vi "AlliGator Get Phasor Ratio Map Color v3.vi"(7 "Color Fading?":bool, 8 "Error In":errorcluster, 9 "Pixel Color":T1, 10 "-d_0":sgl, 11 "Phasor Ratio Data":T2) -> (0 "Error Out":errorcluster, 1 "Transparent?":bool, 3 "Overlay Color":T1)   [LabVIEW 2021, in "AlliGator Phasor Ratio.lvlib"]
doc: "Computes phasor ratio equivalent color using the provided color scale."
uses:
  AlliGator Phasor Ratio.lvlib
  AlliGator Phasor Ratio Data.ctl
panel:
  # "see the AlliGator License on the block diagram (Ctrl+E or Window:Show Block Diagram)"
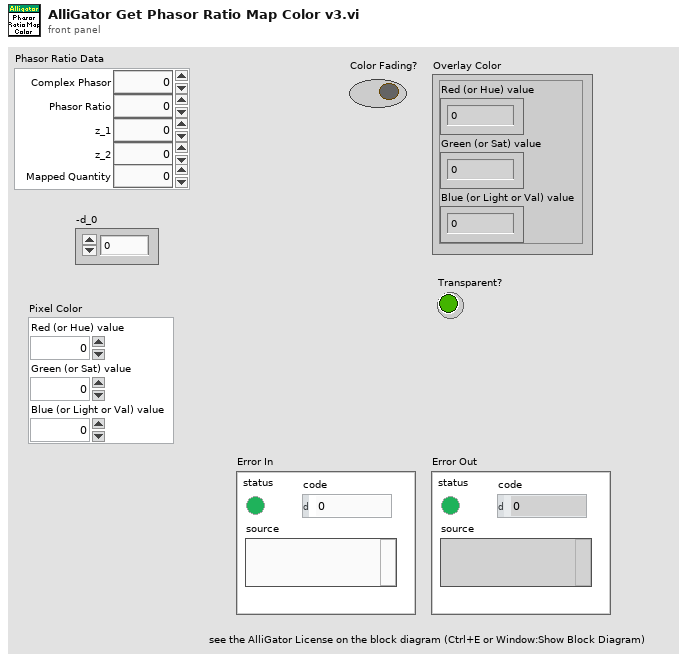
[diagram p1: front panel]
types:
  T1 = cluster{"Red (or Hue) value":u8, "Green (or Sat) value":u8, "Blue (or Light or Val) value":u8}
  T2 = typedef "AlliGator Phasor Ratio.lvlib/AlliGator Phasor Ratio Data.ctl" = cluster{"Complex Phasor":csg, "Phasor Ratio":sgl, "z_1":csg, "z_2":csg, "Mapped Quantity":sgl}
  T3 = cluster{"Red (or Hue) value":sgl, "Green (or Sat) value":sgl, "Blue (or Light or Val) value":sgl}
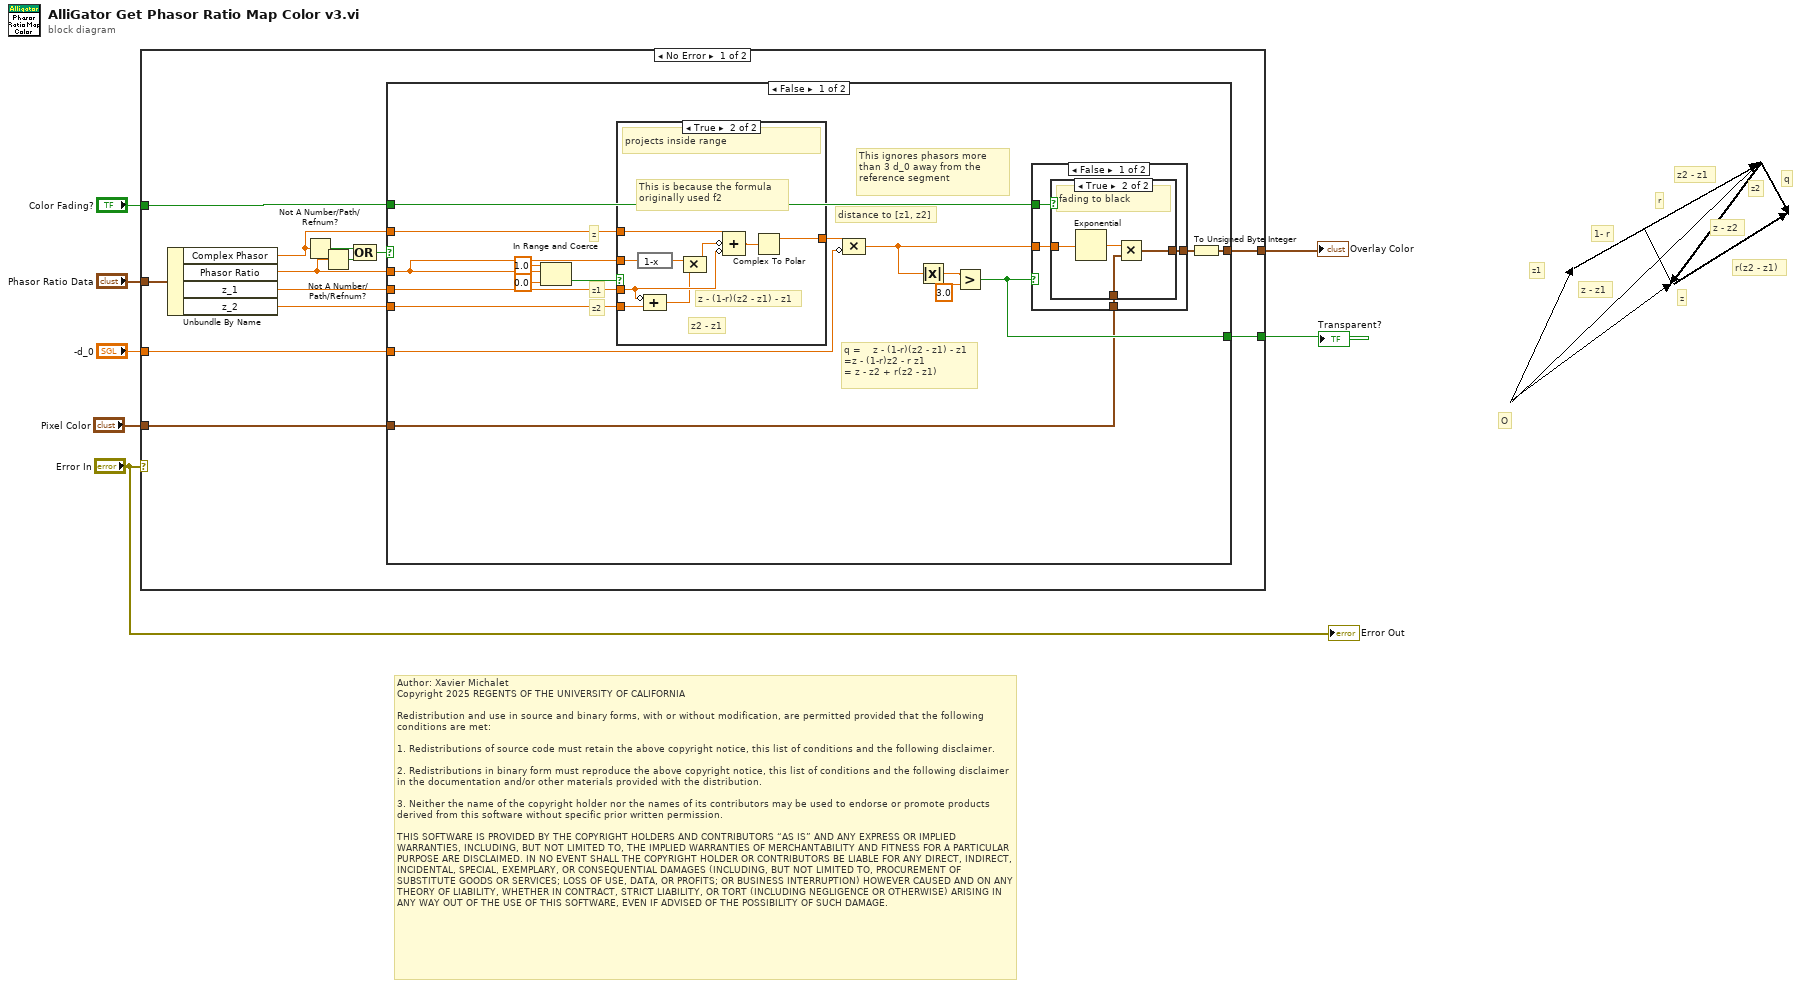
[diagram p0: block diagram]
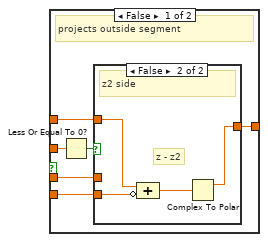
[diagram p4: hidden frame]
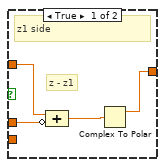
[diagram p5: hidden frame]
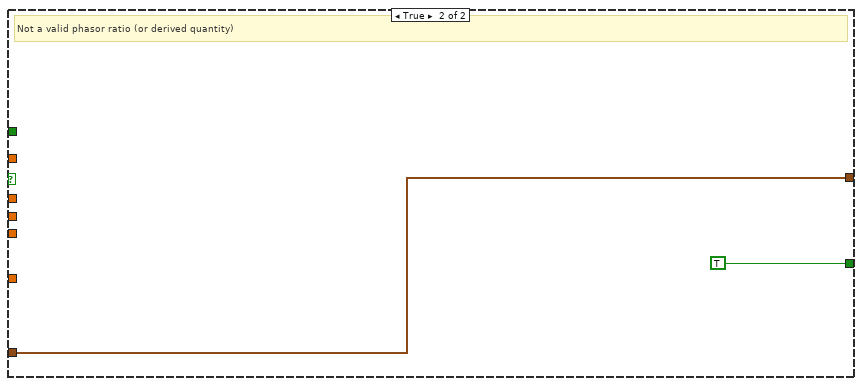
[diagram p6: hidden frame]
diagram:
  # "Author: Xavier Michalet\nCopyright 2025 REGENTS OF THE UNIVERSITY OF CALIFORNIA\n\nRedistribution and use in source and binary forms, with or without modification, are permitted provided that the following conditions are met:\n\n1. Redistributions of source code must retain the above copyright notice, this list of conditions and the following disclaimer.\n\n2. Redistributions in binary form must reproduce the above copyright notice, this list of conditions and the following disclaimer in the documentation and/or other materials provided with the distribution.\n\n3. Neither the name of the copyright holder nor the names of its contributors may be used to endorse or promote products derived from this software without specific prior written permission.\n\nTHIS SOFTWARE IS PROVIDED BY THE COPYRIGHT HOLDERS AND CONTRIBUTORS “AS IS” AND ANY EXPRESS OR IMPLIED WARRANTIES, INCLUDING, BUT NOT LIMITED TO, THE IMPLIED WARRANTIES OF MERCHANTABILITY AND FITNESS FOR A PARTICULAR PURPOSE ARE DISCLAIMED. IN NO EVENT SHALL THE COPYRIGHT HOLDER OR CONTRIBUTORS BE LIABLE FOR ANY DIRECT, INDIRECT, INCIDENTAL, SPECIAL, EXEMPLARY, OR CONSEQUENTIAL DAMAGES (INCLUDING, BUT NOT LIMITED TO, PROCUREMENT OF SUBSTITUTE GOODS OR SERVICES; LOSS OF USE, DATA, OR PROFITS; OR BUSINESS INTERRUPTION) HOWEVER CAUSED AND ON ANY THEORY OF LIABILITY, WHETHER IN CONTRACT, STRICT LIABILITY, OR TORT (INCLUDING NEGLIGENCE OR OTHERWISE) ARISING IN ANY WAY OUT OF THE USE OF THIS SOFTWARE, EVEN IF ADVISED OF THE POSSIBILITY OF SUCH DAMAGE."
  # "O"
  # "q"
  # "r(z2 - z1)"
  # "1- r"
  # "r"
  # "z - z2"
  # "z - z1"
  # "z2 - z1"
  # "z"
  # "z2"
  # "z1"
  n1 = case shown="No Error" "Error In" {
    tunnel: "-d_0" -> [w20 _]
    tunnel: [w19 _] -> w6
    tunnel: [w18 _] -> w5
    tunnel: "Color Fading?" -> [w17 _]
    tunnel: "Phasor Ratio Data" -> [w13 _]
    tunnel: "Pixel Color" -> [w8 _]
    frame No Error {
      n2 = Unbundle By Name(w13) -> ("Complex Phasor"=w12:csg, "Phasor Ratio"=w11:sgl, "z_1"=w10:csg, "z_2"=w9:csg)
      n3 = Not A Number/Path/Refnum?(number/path/refnum=w12) -> (NaN/Path/Refnum?=w16:bool)
      n4 = Not A Number/Path/Refnum?(number/path/refnum=w11) -> (NaN/Path/Refnum?=w15:bool)
      n5 = Compound Arithmetic op=OR(w16, w15) -> (w14:bool)
      n6 = case shown="False" w14 {
        tunnel: w10 -> [w37 _]
        tunnel: w9 -> [w36 _]
        tunnel: w20 -> [w34 _]
        tunnel: [w29 w71] -> w19
        tunnel: [w32 TRUE] -> w18
        tunnel: w17 -> [w31 _]
        tunnel: w12 -> [w30 _]
        tunnel: w11 -> [w28 _]
        tunnel: w8 -> [w21 w71]
        frame False {
          # "distance to [z1, z2]"
          # "q =    z - (1-r)(z2 - z1) - z1\n=z - (1-r)z2 - r z1\n= z - z2 + r(z2 - z1)"
          # "z"
          # "z2"
          # "z1"
          # "This ignores phasors more than 3 d_0 away from the reference segment"
          n7 = In Range and Coerce(upper limit=sgl 1.0, x=w28, lower limit=sgl 0.0) -> (In Range?=w27:bool)  [unwired: 1 out]
          n8 = case shown="True" w27 {
            tunnel: w30 -> [w51 w70]
            tunnel: w37 -> [w50 w64]
            tunnel: w28 -> [w53 w69]
            tunnel: [w49 w66] -> w35
            tunnel: w36 -> [w48 w65]
            frame False {
              # "projects outside segment"
              n9 = Less Or Equal To 0?(x=w53) -> (x <= 0?=w52:bool)
              n10 = case shown="False" w52 {
                tunnel: w51 -> [w57 w61]
                tunnel: w50 -> [w56 _]
                tunnel: [w54 w59] -> w49
                tunnel: w48 -> [_ w58]
                frame True {
                  # "z - z1"
                  # "z1 side"
                  n11 = Compound Arithmetic op=ADD(w57, invert w56) -> (w55:csg)
                  n12 = Complex To Polar(r * e^(i*theta)=w55) -> (r=w54:sgl)  [unwired: 1 out]
                }
                frame False {
                  # "z - z2"
                  # "z2 side"
                  n13 = Compound Arithmetic op=ADD(w61, invert w58) -> (w60:csg)
                  n14 = Complex To Polar(r * e^(i*theta)=w60) -> (r=w59:sgl)  [unwired: 1 out]
                }
              }
            }
            frame True {
              # "z - (1-r)(z2 - z1) - z1"
              # "z2 - z1"
              # "This is because the formula originally used f2"
              # "projects inside range"
              n15 = expression code="1-x"(w69) -> (w62:sgl)
              n16 = Compound Arithmetic op=ADD(invert w64, w65) -> (w63:csg)
              n17 = Compound Arithmetic op=MULTIPLY(w62, w63) -> (w68:csg)
              n18 = Compound Arithmetic op=ADD(w70, invert w68, invert w64) -> (w67:csg)
              n19 = Complex To Polar(r * e^(i*theta)=w67) -> (r=w66:sgl)  [unwired: 1 out]
            }
          }
          n20 = Compound Arithmetic op=MULTIPLY(w35, invert w34) -> (w24:sgl)
          n21 = Absolute Value(x=w24) -> (abs(x)=w23:sgl)
          n22 = Greater?(x=w23, y=sgl 3.0) -> (0:w32:bool)
          n23 = case shown="False" w32 {
            tunnel: w21 -> [w41 w47]
            tunnel: w24 -> [w40 _]
            tunnel: [w39 w47] -> w33
            tunnel: w31 -> [w38 _]
            frame False {
              n24 = case shown="True" w38 {
                tunnel: w41 -> [w42 w46]
                tunnel: w40 -> [_ w44]
                tunnel: [w42 w43] -> w39
                frame False {
                }
                frame True {
                  # "fading to black"
                  n25 = Exponential(1:w44) -> (0:w45:sgl)
                  n26 = Multiply(x=w45, y=w46) -> (x*y=w43:T3)
                }
              }
            }
            frame True {
            }
          }
          n27 = To Unsigned Byte Integer(number=w33) -> (unsigned 8bit integer=w29:T1)
        }
        frame True {
          # "Not a valid phasor ratio (or derived quantity)"
        }
      }
    }
    frame Error {
    }
  }
  "Overlay Color" <- w6
  "Transparent?" <- w5
  "Error Out" <- "Error In"
